vi "fcs plot.vi"(9 "par2":i32, 10 "par1":i32, 11 "Array in":sgl[][](array[numeric])) -> (2 "par1 plot":sgl[](array[numeric]), 3 "xy plot":cluster{"Array":sgl[], "Array":sgl[]})   [LabVIEW 2013]
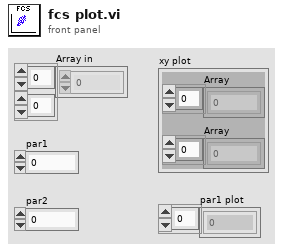
[diagram p1: front panel]
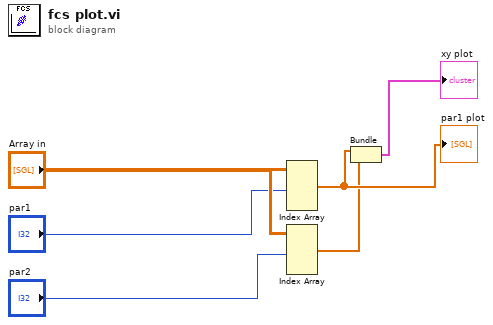
[diagram p0: block diagram]
diagram:
  n1 = Index Array(array="Array in", index (col) #1="par1") -> (element #1=w5:sgl[])  [unwired: 3 in, 1 out]
  "par1 plot" <- w5
  n2 = Index Array(array="Array in", index (col) #1="par2") -> (element #1=w3:sgl[])  [unwired: 3 in, 1 out]
  n3 = Bundle("Array in"=w5, "Array in"=w3) -> (→"xy plot":cluster{"Array in":sgl[], "Array in":sgl[]})  [unwired: 1 in]
